vi "GetLimits.vi"(8 "error in (no error)":errorcluster, 10 "Axis":T1 items=["1"=1, "2"=2, "3"=3, "4"=4], 11 "DLOwis in":refnum<class "DLOwis.lvclass">) -> (0 "error out":errorcluster, 1 "max":dbl, 2 "min":dbl, 3 "DLOwis out":refnum<class "DLOwis.lvclass">, 4 "real pos, mm":dbl)   [LabVIEW 2019]
uses:
  DelayLineLS4/LS4 axis.ctl
  DelayLine.lvclass
  DLOwis.lvclass
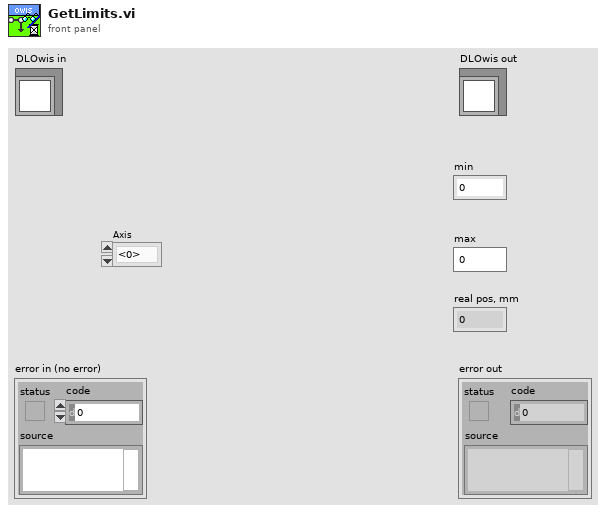
[diagram p1: front panel]
types:
  T1 = typedef "DelayLine.lvclass/LS4 axis.ctl" = u16
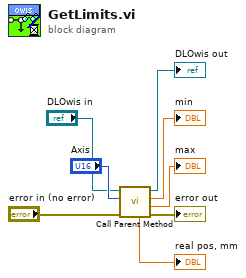
[diagram p0: block diagram]
diagram:
  n1 = call-parent "Call Parent Method"("error in (no error)"="error in (no error)", "Axis"="Axis", "DelayLine in"="DLOwis in") -> ("error out"=→"error out":errorcluster, "max"=→"max":dbl, "min"=→"min":dbl, "DelayLine out"=→"DLOwis out":refnum<class "DLOwis.lvclass">, "real pos, mm"=→"real pos, mm":dbl)  [unwired: 4 in]
